vi "Add_Shear_Ramp_Job.vi"(7 "New Job":bool=TRUE, 8 "error in (no error)":errorcluster, 9 "Tag Item":string, 10 "ShearRampConfiguration":T1={"Shear Ramp"="Linear", "Rotation or Torque"="", "Initial Value"=0.0, "Final Value"=0.0, "Duration"=0.0, "Number of Points"=0, "Confirmed?"=FALSE, "Shear Ramp Array"=[]}, 11 "TreeControl in":refnum<vi>) -> (0 "error out":errorcluster)   [LabVIEW 2021]
uses:
  TypeDefs/ShearRampConfiguration.ctl
panel:
  out "Job Attributes":string
  out "TreeControl out":refnum<vi>
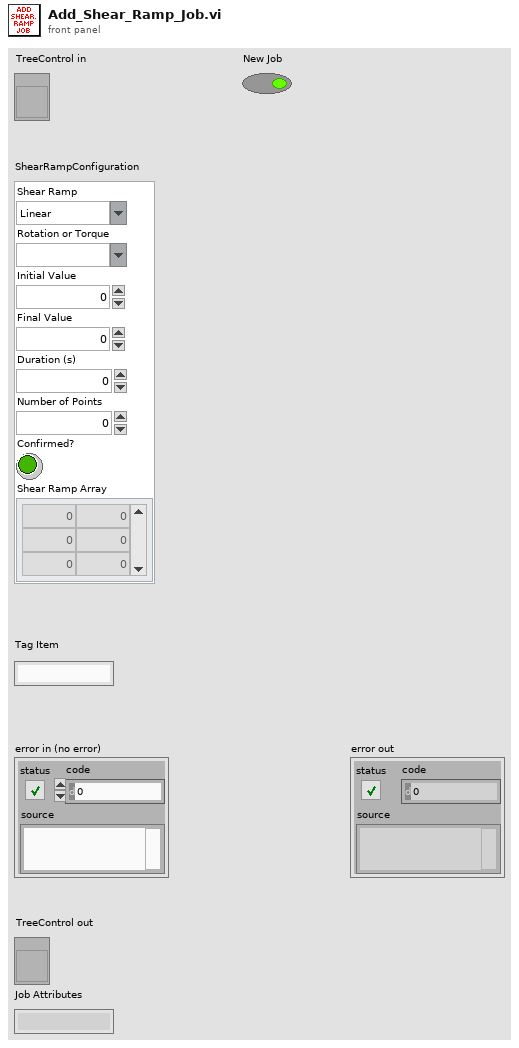
[diagram p1: front panel]
types:
  T1 = typedef "ShearRampConfiguration.ctl" = cluster{"Shear Ramp":string, "Rotation or Torque":string, "Initial Value":dbl, "Final Value":dbl, "Duration":dbl, "Number of Points":i32, "Confirmed?":bool, "Shear Ramp Array":dbl[][]}
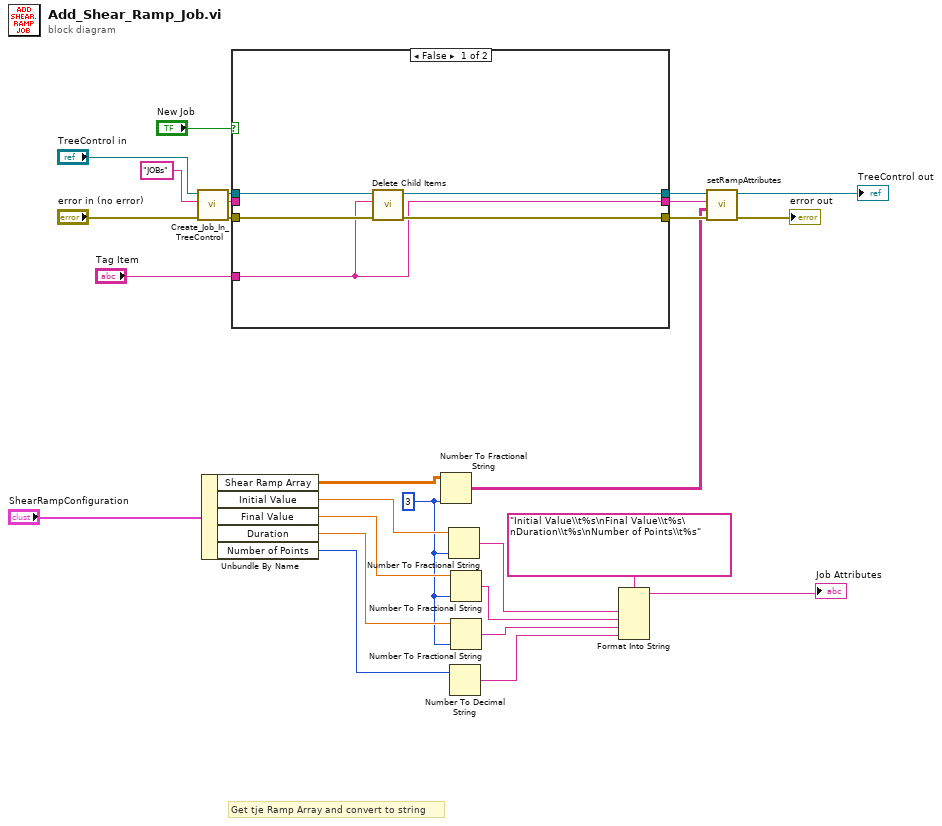
[diagram p0: block diagram]
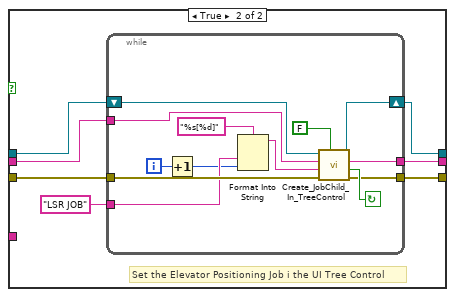
[diagram p2: hidden frame]
diagram:
  w4 = i16 3 ("precision (6)")
  # "Get tje Ramp Array and convert to string"
  n1 = call "Create_Job_In_TreeControl.vi"("error in (no error)"="error in (no error)", "Left Cell String"="JOBs", "TreeControl in"="TreeControl in") -> ("error out"=w23:errorcluster, "Edit Tree Items:Add Item"=w26:string, "TreeControl out"=w27:refnum<vi>)  [unwired: 6 in]
  n2 = Unbundle By Name("ShearRampConfiguration") -> ("Shear Ramp Array"=w3:dbl[][], "Initial Value"=w15:dbl, "Final Value"=w14:dbl, "Duration"=w12:dbl, "Number of Points"=w13:i32)
  n3 = case shown="False" "New Job" {
    tunnel: w27 -> [w32 w39]
    tunnel: w26 -> [_ w38]
    tunnel: w23 -> [w31 w36]
    tunnel: [w30 w35] -> w20
    tunnel: [w29 w34] -> w19
    tunnel: [w28 w33] -> w18
    tunnel: "Tag Item" -> [w29 _]
    frame False {
      n4 = call "Delete Child Items.vi"("error in (no error)"=w31, "Item Edit"=w29, "TreeControl in"=w32) -> ("error out"=w30:errorcluster, "TreeControl out"=w28:refnum<vi>)  [unwired: 7 in]
    }
    frame True {
      # "Set the Elevator Positioning Job i the UI Tree Control"
      n5 = while {
        tunnel: w36 -> [w52]
        tunnel: "LSR JOB" -> [w41]
        tunnel: w38 -> [w49]
        tunnel: [w44] -> w35
        tunnel: [w43] -> w34
        shift-right: [w42] -> w33
        shift-left: w39 -> [w48]
        i -> [w46]
        stop <- w45 continue-if-true
        n6 = Increment(x=w46) -> (x+1=w40:i32)
        n7 = Format Into String(format string="%s[%d]", w41, w40) -> (resulting string=w50:string)  [unwired: 2 in, 1 out]
        n8 = call "Create_JobChild_In_TreeControl.vi"("Child Only?"=FALSE, "error in (no error)"=w52, "Child Tag Name"=w50, "Parent Item"=w49, "TreeControl in"=w48) -> ("error out"=w44:errorcluster, "Tag Already Exists?"=w45:bool, "Edit Tree Items:Add Item 2"=w43:string, "TreeControl out"=w42:refnum<vi>)  [unwired: 3 in]
      }
    }
  }
  n9 = Number To Fractional String(number=w3, precision (6)=w4) -> (F-format string=w5:string[][])  [unwired: 2 in]
  n10 = Number To Fractional String(number=w15, precision (6)=w4) -> (F-format string=w10:string)  [unwired: 2 in]
  n11 = Number To Decimal String(number=w13) -> (decimal integer string=w7:string)  [unwired: 1 in]
  n12 = Number To Fractional String(number=w14, precision (6)=w4) -> (F-format string=w9:string)  [unwired: 2 in]
  n13 = Number To Fractional String(number=w12, precision (6)=w4) -> (F-format string=w8:string)  [unwired: 2 in]
  n14 = Format Into String(format string="Initial Value\\t%s\nFinal Value\\t%s\nDuration\\t%s\nNumber of Points\\t%s", w10, w9, w8, w7) -> (resulting string=→"Job Attributes":string)  [unwired: 2 in, 1 out]
  n15 = call "setRampAttributes.vi"("error in (no error)"=w20, "Array"=w5, "Edit Tree Items:Add Item in"=w19, "TreeControl in"=w18) -> ("error out"=→"error out":errorcluster, "TreeControl out"=→"TreeControl out":refnum<vi>)  [unwired: 6 in]
